vi "Configure Histogram Analysis.vi"(6 "Histogram Size (1)":i32=1, 7 "Histogram Source (0: Channel 1)":u16(ring) items=["Channel 1", "Channel 2", "Channel 3", "Channel 4", "Math 1", "Math 2", "Math 3", "Math 4", "Reference Waveform 1", "Reference Waveform 2", "Reference Waveform 3", "Reference Waveform 4", "Color Grade", "Measurement 1", "Measurement 2", "Measurement 3", "Measurement 4", "Measurement 5", "Measurement 6", "Measurement 7", "Measurement 8", "Measurement 9", "Measurement 10"], 8 "error in (no error)":errorcluster, 9 "Enable Histogram (T: Enable)":bool=TRUE, 10 "Histogram Type (0: Vertical)":i32(ring) items=["Vertical", "Horizontal", "Measurement"], 11 "VISA resource name":refnum<visa-resource-name>) -> (0 "error out":errorcluster, 3 "VISA resource name out":refnum<visa-resource-name>)   [LabVIEW 2023, in "Keysight-DSQx3014T.lvlib"]
doc: "Configures the histogram analysis feature.\n\n<b>Note:</b>\nThis VI is specific to the 6000-X Series oscilloscopes. These features are not available on other models."
uses:
  Keysight-DSQx3014T.lvlib
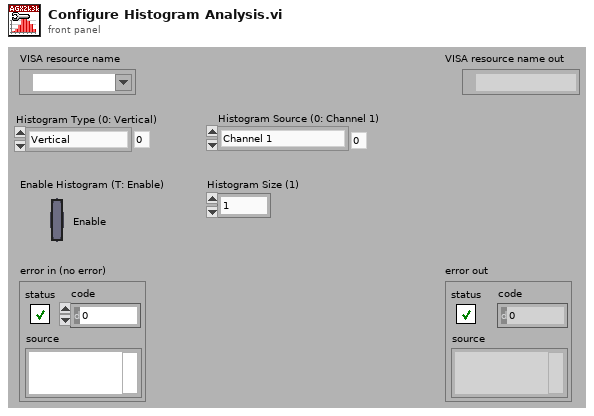
[diagram p1: front panel]
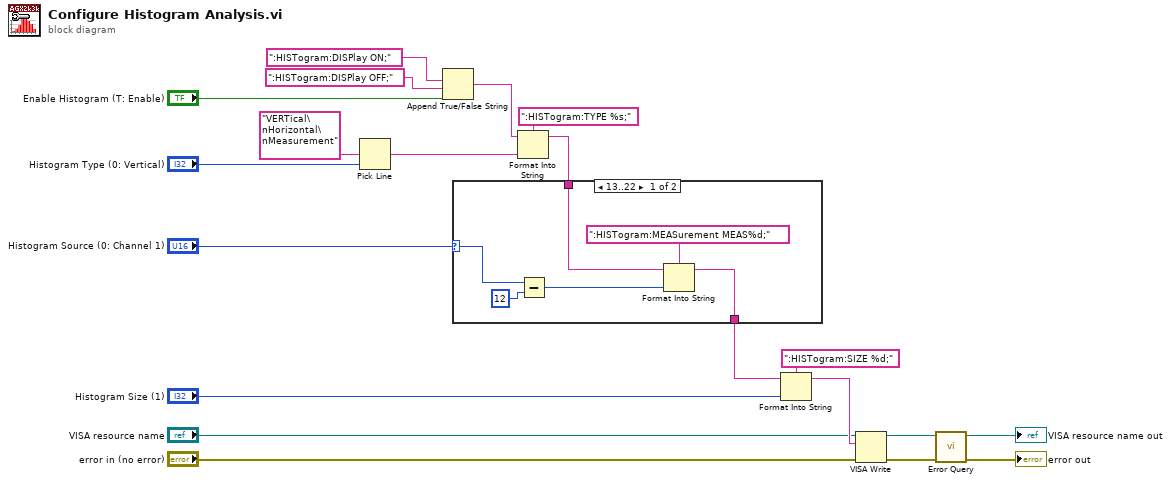
[diagram p0: block diagram]
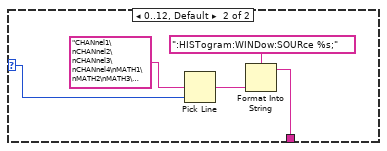
[diagram p2: hidden frame]
diagram:
  n1 = Pick Line(multi-line string="VERTical\nHorizontal\nMeasurement", line index="Histogram Type (0: Vertical)") -> (output string=w9:string)  [unwired: 1 in]
  n2 = Append True/False String(1:"Enable Histogram (T: Enable)", 2:":HISTogram:DISPlay OFF;", 3:":HISTogram:DISPlay ON;") -> (0:w17:string)  [unwired: 1 in]
  n3 = Format Into String(format string=":HISTogram:TYPE %s;", initial string=w17, w9) -> (resulting string=w7:string)  [unwired: 1 in, 1 out]
  n4 = case shown="13..22" "Histogram Source (0: Channel 1)" {
    selector: "Histogram Source (0: Channel 1)" -> [w25 w27]
    tunnel: [w24 w28] -> w6
    tunnel: w7 -> [w21 _]
    frame 13..22 {
      n5 = Subtract(x=w25, y=u16 12) -> (x-y=w23:u16)
      n6 = Format Into String(format string=":HISTogram:MEASurement MEAS%d;", initial string=w21, w23) -> (resulting string=w24:string)  [unwired: 1 in, 1 out]
    }
    frame 0..12, Default {
      n7 = Pick Line(multi-line string="CHANnel1\nCHANnel2\nCHANnel3\nCHANnel4\nMATH1\nMATH2\nMATH3\nMATH4\nWMEMory1\nWMEMory2\nWMEMory3\nWMEMory4\nCGRade", line index=w27) -> (output string=w31:string)  [unwired: 1 in]
      n8 = Format Into String(format string=":HISTogram:WINDow:SOURce %s;", w31) -> (resulting string=w28:string)  [unwired: 2 in, 1 out]
    }
  }
  n9 = Format Into String(format string=":HISTogram:SIZE %d;", initial string=w6, "Histogram Size (1)") -> (resulting string=w13:string)  [unwired: 1 in, 1 out]
  n10 = VISA Write(VISA resource name="VISA resource name", write buffer=w13, error in (no error)="error in (no error)") -> (VISA resource name out=w4:refnum<visa-resource-name>, error out=w3:errorcluster)  [unwired: 1 out]
  n11 = call "Error Query.vi"("error in (no error)"=w3, "VISA resource name"=w4) -> ("error out"=→"error out":errorcluster, "VISA resource name out"=→"VISA resource name out":refnum<visa-resource-name>)  [unwired: 6 in, 2 out]
